vi "Configure Hardware.vi"(8 "error in (no error)":errorcluster caption="错误输入（无错误）", 11 "Hardware Resources in":T1 caption="硬件资源输入") -> (0 "error out":errorcluster caption="错误输出", 3 "Hardware Resources out":T1 caption="硬件资源输出")   [LabVIEW 2014]
doc: "配置硬件。"
uses:
  Hardware Configures.ctl
  <vilib>/DAQmx/create/channels.llb/DAQmx Create Channel (AO-Voltage-Basic).vi
  <vilib>/DAQmx/configure/timing.llb/DAQmx Timing (Sample Clock).vi
  HardWareConfig.lvlib
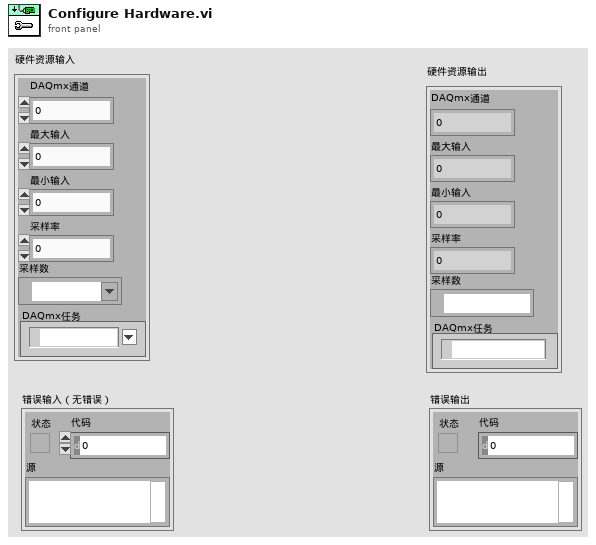
[diagram p1: front panel]
types:
  T1 = typedef "HardWareConfig.lvlib/Hardware Configures.ctl" = cluster{"Max Input":dbl, "Min Input":dbl, "Sample Rate":dbl, "Sample Num":dbl, "DAQmx Task":refnum<k21>, "物理通道":tag}
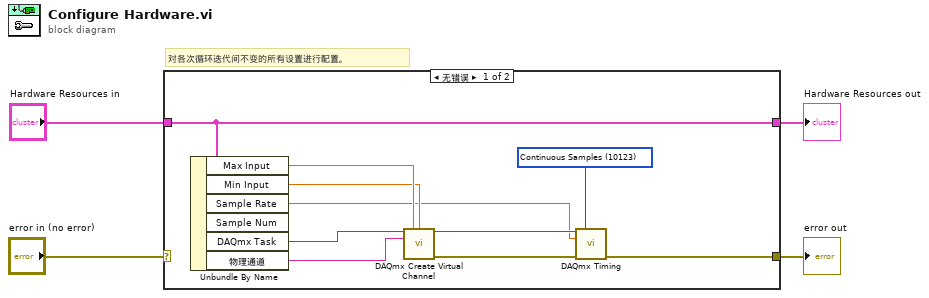
[diagram p0: block diagram]
diagram:
  # "对各次循环迭代间不变的所有设置进行配置。"
  n1 = case shown="无错误" "error in (no error)" {
    selector: "error in (no error)" -> [_ w15]
    tunnel: [w11 w15] -> w3
    tunnel: "Hardware Resources in" -> [w10 w16]
    tunnel: [w10 w16] -> w1
    frame No Error {
      w12 = 10123 items=["Finite Samples"=10178, "Continuous Samples"=10123, "Hardware Timed Single Point"=12522] ("sample mode")
      n2 = Unbundle By Name(w10) -> ("Max Input"=w7:dbl, "Min Input"=w6:dbl, "Sample Rate"=w5:dbl, "DAQmx Task"=w8:refnum<k21>, "物理通道"=w9:tag)  [unwired: 1 out]
      n3 = call-poly <vilib>:"DAQmx Create Virtual Channel.vi"("task in"=w8, "maximum value"=w7, "minimum value"=w6, "physical channels"=w9) -> ("task out"=w14:refnum<k21>, "error out"=w13:errorcluster)  [unwired: 10 in]
      n4 = call-poly <vilib>:"DAQmx Timing.vi"("task/channels in"=w14, "sample mode"=w12, "rate"=w5, "error in"=w13) -> ("error out"=w11:errorcluster)  [unwired: 10 in, 1 out]
    }
    frame Error {
    }
  }
  "Hardware Resources out" <- w1
  "error out" <- w3
